vi "Copy Library Item.vi"(8 "error in (no error)":errorcluster, 9 "Copy Name":string, 10 "Copy location":path, 11 "Library in":refnum<vi>) -> (0 "error out":errorcluster, 2 "New Lib Path":path, 3 "Library out":refnum<vi>)   [LabVIEW 2019, in "gRPC Template Creation Utility.lvlib"]
uses:
  gRPC Template Creation Utility.lvlib
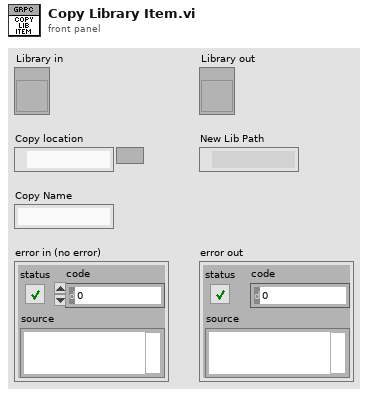
[diagram p1: front panel]
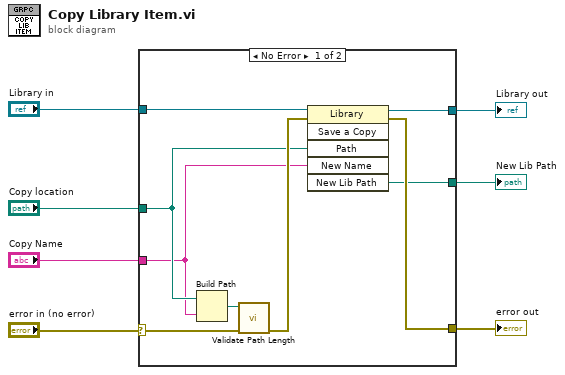
[diagram p0: block diagram]
diagram:
  n1 = case shown="No Error" "error in (no error)" {
    selector: "error in (no error)" -> [w8 w17]
    tunnel: [w15 w18] -> w7
    tunnel: [w14 w17] -> w6
    tunnel: "Library in" -> [w13 w18]
    tunnel: [w12 _] -> w4
    tunnel: "Copy Name" -> [w10 _]
    tunnel: "Copy location" -> [w11 _]
    frame No Error {
      n2 = Build Path(base path=w11, name or relative path=w10) -> (appended path=w9:path)
      n3 = call "Validate Path Length.vi"("error in (no error)"=w8, "Path in"=w9) -> ("error out"=w16:errorcluster)  [unwired: 8 in, 1 out]
      n4 = invoke class="Library" method="Save a Copy"(reference=w13, error in=w16, "Path"=w11, "New Name"=w10) -> (reference out=w15:refnum<vi>, error out=w14:errorcluster, "New Lib Path"=w12:path)  [unwired: 2 in, 3 out]
    }
    frame Error {
    }
  }
  "Library out" <- w7
  "error out" <- w6
  "New Lib Path" <- w4
